vi "ps5000a acquire GEECS.vi"(8 "Error in":errorcluster, 11 "Picoscope in":refnum<class "picoscope.lvclass">) -> (0 "Error out":errorcluster, 1 "GEECS waveforms info":T3(array[cluster]), 2 "TraceGUI-Info":T2, 3 "scope traces":i16[][](array[numeric]), 4 "Channel A Settings":T1, 5 "Waveforms":waveform(dbl)[](graph), 6 "Picoscope out":refnum<class "picoscope.lvclass">)   [LabVIEW 2020, in "picoscope.lvclass"]
uses:
  picoscope.lvclass
  TraceGUI-Info.ctl
  picoscope.lvclass/picoscope.ctl
panel:
  out "Channel B Settings":T1
  out "time (ms)":u32
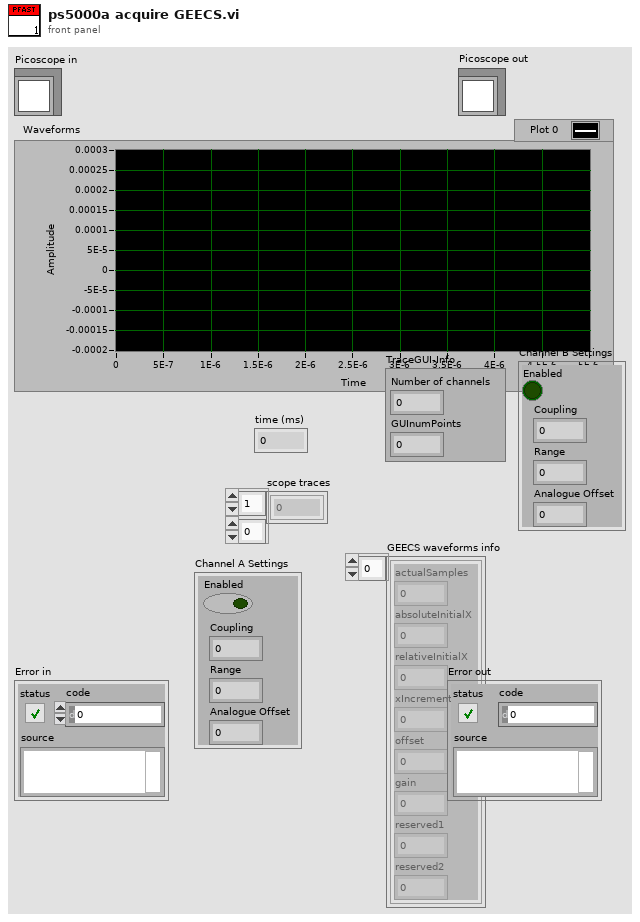
[diagram p1: front panel]
types:
  T1 = cluster{"Enabled":bool, "Coupling":i16, "Range":u16, "Analogue Offset":sgl}
  T2 = typedef "TraceGUI-Info.ctl" = cluster{"Number of channels":dbl, "GUInumPoints":i32}
  T3 = cluster{"actualSamples":i32, "absoluteInitialX":dbl, "relativeInitialX":dbl, "xIncrement":dbl, "offset":dbl, "gain":dbl, "reserved1":dbl, "reserved2":dbl}[]
  T4 = cluster{"Driver Version":string, "USB Version":string, "Hardware":string, "Variant":string, "Batch and Serial":string, "Cal Date":string, "Kernel Version":string, "Digital HW Version":string, "Analogue HW Version":string, "MSO":bool, "Number of channels":i16}
  T5 = cluster{"preTriggerSamples":u32, "postTriggerSamples":u32, "timebase":u32, "Down-Sample Mode":i32, "Down Sample Ratio":u32, "Number of Captures":u32}
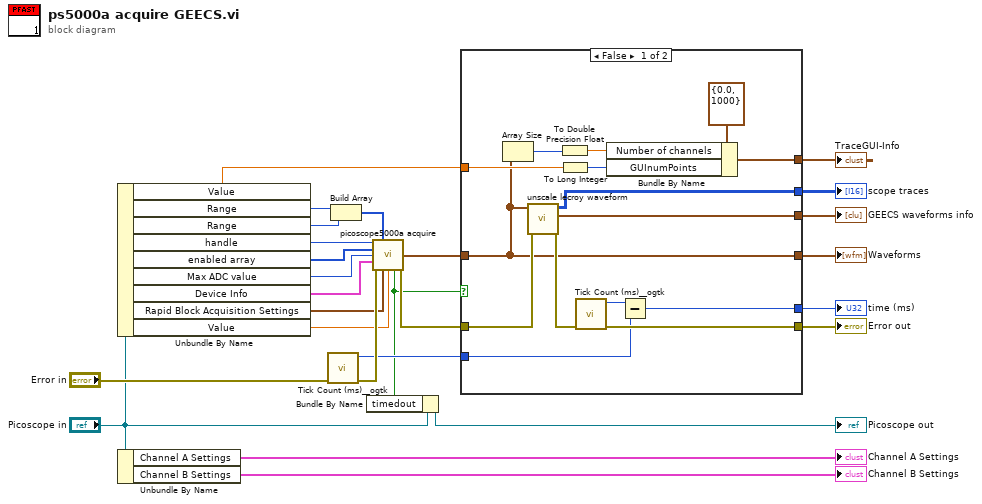
[diagram p0: block diagram]
diagram:
  n1 = Unbundle By Name("Picoscope in") -> ("Value"=w12:dbl, "Range"=w22:u16, "Range"=w13:u16, "handle"=w18:i16, "enabled array"=w24:i16[], "Max ADC value"=w19:i16, "Device Info"=w20:T4, "Rapid Block Acquisition Settings"=w23:T5, "Value"=w14:dbl)
  n2 = Unbundle By Name("Picoscope in") -> ("Channel A Settings"=→"Channel A Settings":T1, "Channel B Settings"=→"Channel B Settings":T1)
  n3 = call "Tick Count (ms)__ogtk.vi"("error in (no error)"="Error in") -> ("error out"=w26:errorcluster, "millisecond timer value"=w15:u32)  [unwired: 9 in]
  n4 = Build Array(w22, w13) -> (w25:u16[])
  n5 = call "picoscope5000a acquire.vi"("handle in"=w18, "Ranges"=w25, "enabled array"=w24, "Max ADC value"=w19, "Device Info"=w20, "error in (no error)"=w26, "Rapid Block Acquisition Settings"=w23, "timeout"=w14) -> ("Waveform Data"=w21:waveform(dbl)[], "timedout"=w1:bool, "error out"=w16:errorcluster)  [unwired: 2 in, 3 out]
  n6 = Bundle By Name(cluster="Picoscope in", "timedout"=w1) -> (→"Picoscope out":refnum<class "picoscope.lvclass">)
  n7 = case shown="False" w1 {
    tunnel: w21 -> [w32 _]
    tunnel: w12 -> [w40 _]
    tunnel: w16 -> [w34 w42]
    tunnel: w15 -> [w36 _]
    tunnel: [w41 w42] -> w10
    tunnel: [w35 _] -> w9
    tunnel: [w32 _] -> w8
    tunnel: [w31 _] -> w7
    tunnel: [w30 _] -> w6
    tunnel: [w29 _] -> w5
    frame False {
      n8 = Array Size(array=w32) -> (size(s)=w39:i32)
      n9 = call "unscale lecroy waveform.vi"("Error in"=w34, "Waveforms"=w32) -> ("Error out"=w33:errorcluster, "GEECS waveforms info"=w35:T3, "scope traces"=w30:i16[][])  [unwired: 7 in]
      n10 = To Double Precision Float(number=w39) -> (double precision float=w28:dbl)
      n11 = To Long Integer(number=w40) -> (32bit integer=w27:i32)
      n12 = call "Tick Count (ms)__ogtk.vi"("error in (no error)"=w33) -> ("error out"=w41:errorcluster, "millisecond timer value"=w37:u32)  [unwired: 9 in]
      n13 = Bundle By Name(cluster=T2 {"Number of channels"=0.0, "GUInumPoints"=1000} ("TraceGUI-Info"), "Number of channels"=w28, "GUInumPoints"=w27) -> (w29:T2)
      n14 = Subtract(x=w37, y=w36) -> (x-y=w31:u32)
    }
    frame True {
    }
  }
  "Error out" <- w10
  "GEECS waveforms info" <- w9
  "Waveforms" <- w8
  "time (ms)" <- w7
  "scope traces" <- w6
  "TraceGUI-Info" <- w5
